vi "q2 equation.vi"() -> ()   [LabVIEW 2025]
panel:
  out "y":dbl
  in  "b":dbl
  in  "a":dbl
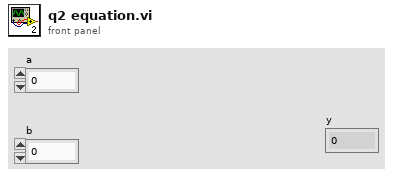
[diagram p1: front panel]
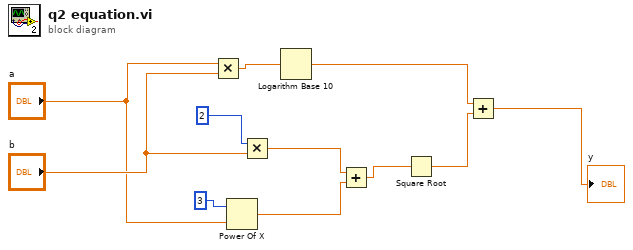
[diagram p0: block diagram]
diagram:
  n1 = Multiply(x="a", y="b") -> (x*y=w11:dbl)
  n2 = Power Of X(1:"a", 2:3) -> (0:w5:dbl)
  n3 = Multiply(x=2, y="b") -> (x*y=w6:dbl)
  n4 = Logarithm Base 10(1:w11) -> (0:w2:dbl)
  n5 = Add(x=w6, y=w5) -> (x+y=w4:dbl)
  n6 = Square Root(x=w4) -> (sqrt(x)=w3:dbl)
  n7 = Add(x=w2, y=w3) -> (x+y=→"y":dbl)
